vi "PH_gentec_Powermeter.Action set Settings.vi"(0 "VI in":refnum<vi>, 5 "error in (no error)":errorcluster) -> (14 "VI out":refnum<vi>, 19 "error out":errorcluster)   [LabVIEW 2014, in "PH_gentec_Powermeter.lvlib"]
uses:
  PH_gentec_Powermeter.lvlib
  PH_Powermeter_BaseClass/PH_Powermeter_BaseClass.State.ctl
  PH_Powermeter_BaseClass/PH_Powermeter_BaseClass.lvlib
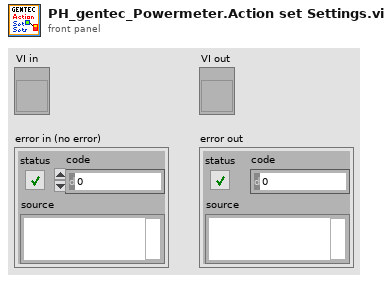
[diagram p1: front panel]
types:
  T1 = typedef "PH_Powermeter_BaseClass.lvlib/PH_Powermeter_BaseClass.State.ctl" = enum32{"off", "operating", "opened", "checked", "connected", "Sets to change", "running"}
  T2 = typedef "PH_Powermeter_BaseClass.lvlib/PH_Powermeter_BaseClass.i attribute.ctl" = cluster{"GUI References":T3, "Connection":T4, "Head Attributes":T5, "VISA resource":refnum<visa-resource-name>, "Energy":T6, "Service ID Energy":i32, "Wanted Settings":T7, "Current Settings":T7}
  T3 = typedef "PH_Powermeter_BaseClass.lvlib/PH_Powermeter_BaseClass.GUI Refs.ctl" = cluster{"Head Attributes":refnum<vi>, "Energy":refnum<vi>, "Connection":refnum<vi>, "VISA Resource":refnum<vi>, "Energy evolution":refnum<vi>, "Scaling Factor":refnum<vi>, "Range":refnum<vi>, "Wavelength":refnum<vi>, "Trigger Level":refnum<vi>, "Wanted Settings":refnum<vi>, "Current Settings":refnum<vi>}
  T4 = typedef "PH_Powermeter_BaseClass.lvlib/PH_Powermeter_BaseClass.Connection.ctl" = cluster{"failed checks":i8, "Timeout":bool, "Data read":string, "Failure":bool, "Error":bool, "State":T1}
  T5 = typedef "PH_Powermeter_BaseClass.lvlib/PH_Powermeter_BaseClass.Head Attributes.ctl" = cluster{"Instrument Type":string, "Head Version":string, "Head Name":string, "Serial Number":string, "Firmware":string, "Sensor Type":string, "MinimumRange":u32, "Maximum Range":u32, "Min Wavelength":i32, "Max Wavelength":i32}
  T6 = typedef "PH_Powermeter_BaseClass.lvlib/PH_Powermeter_BaseClass.Energy.ctl" = cluster{"current Value":dbl, "unscaled":dbl, "Scaling Factor":dbl}
  T7 = typedef "PH_Powermeter_BaseClass.lvlib/PH_gentec_BaseClass.Head Settings.ctl" = cluster{"Trigger Level":dbl, "Wavelength":u32, "Range":u32}
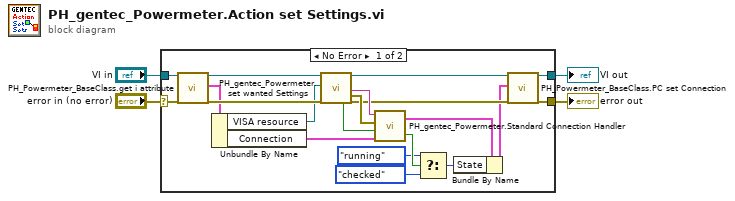
[diagram p0: block diagram]
diagram:
  n1 = case shown="No Error" "error in (no error)" {
    selector: "error in (no error)" -> [w5 w25]
    tunnel: "VI in" -> [w19 w26]
    tunnel: [w13 w25] -> w2
    tunnel: [w10 w26] -> w3
    frame No Error {
      n2 = call "PH_Powermeter_BaseClass.get i attribute.vi"("i ref in"=w19, "error in (no error)"=w5) -> ("i ref out"=w18:refnum<vi>, "i attribute"=w17:T2, "error out"=w20:errorcluster)  [unwired: 15 in]
      n3 = Unbundle By Name(w17) -> ("VISA resource"=w16:refnum<visa-resource-name>, "Connection"=w15:T4)
      n4 = call "PH_gentec_Powermeter.set wanted Settings.vi"("i ref in"=w18, "VISA resource in"=w16, "error in"=w20) -> ("Timeout"=w21:bool, "i ref out"=w11:refnum<vi>, "Error Messages"=w24:string, "Device Error out"=w23:errorcluster, "error out"=w14:errorcluster)  [unwired: 12 in]
      n5 = call "PH_gentec_Powermeter.Standard Connection Handler.vi"("Connection in"=w15, "Timeout"=w21, "Device Error"=w23, "Error"=w24) -> ("No problem"=w9:bool, "Connection out"=w22:T4)
      n6 = Select(t=PH_Powermeter_BaseClass.State."running" ("State"), s=w9, f=PH_Powermeter_BaseClass.State."checked") -> (s? t:f=w7:T1)
      n7 = Bundle By Name(cluster=w22, "State"=w7) -> (w12:T4)
      n8 = call "PH_Powermeter_BaseClass.PC set Connection.vi"("VI in"=w11, "Connection"=w12, "error in (no error)"=w14) -> ("VI out"=w10:refnum<vi>, "error out"=w13:errorcluster)  [unwired: 15 in]
    }
    frame Error {
    }
  }
  "VI out" <- w3
  "error out" <- w2
